vi "SetValue.vi"(0 "class data in":refnum<class "AbruptChange.lvclass">, 5 "Value":dbl, 11 "error in (no error)":errorcluster) -> (4 "class data out":refnum<class "AbruptChange.lvclass">, 15 "error out":errorcluster)   [LabVIEW 2019, in "AbruptChange.lvclass"]
uses:
  AbruptChange.lvclass
  AbruptChange.lvclass/AbruptChange.ctl
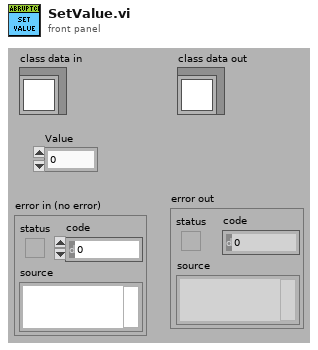
[diagram p1: front panel]
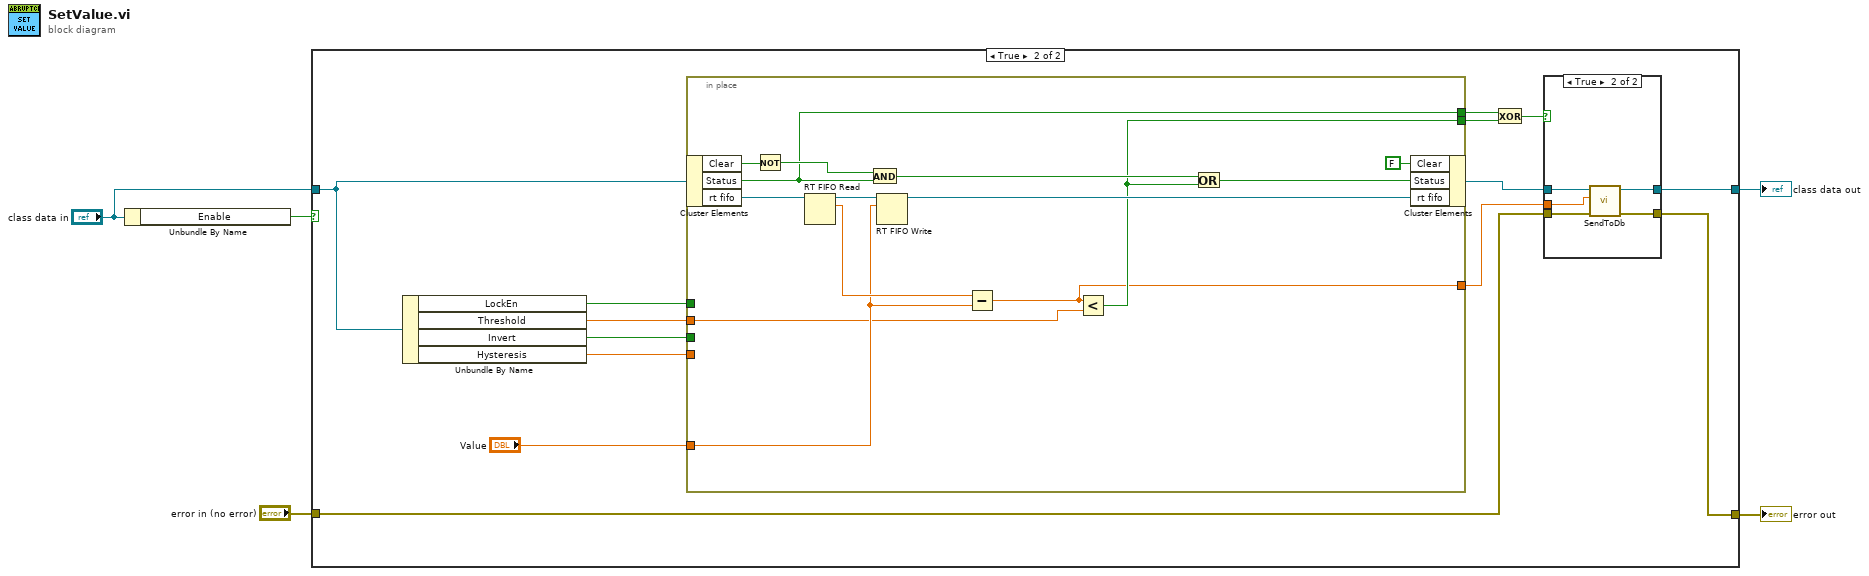
[diagram p0: block diagram]
diagram:
  n1 = Unbundle By Name("class data in") -> ("Enable"=w4:bool)
  n2 = case shown="True" w4 {
    tunnel: [w7 w15] -> w5
    tunnel: "class data in" -> [w7 w21]
    tunnel: "error in (no error)" -> [w6 w14]
    tunnel: [w6 w13] -> w1
    frame False {
    }
    frame True {
      n3 = Unbundle By Name(w21) -> ("LockEn"=w17:bool, "Threshold"=w19:dbl, "Invert"=w18:bool, "Hysteresis"=w20:dbl)
      n4 = in-place {
        in-place-border: w19 -> [w38]
        in-place-border: w20 -> [_]
        in-place-border: w18 -> [_]
        in-place-border: w17 -> [_]
        in-place-border: "Value" -> [w39]
        in-place-border: [w31] -> w10
        in-place-border: [w30] -> w9
        in-place-border: [w29] -> w8
        n5 = in-place-cluster #1(w21) -> ("Clear"=w34:bool, "Status"=w30:bool, "rt fifo"=w42:refnum<k33>)
        n6 = Not(x=w34) -> (.not. x?=w35:bool)
        n7 = RT FIFO Read(0:w42) -> (8:w41:refnum<k33>, 9:w40:dbl)  [unwired: 3 in, 3 out]
        n8 = And(x=w35, y=w30) -> (x .and. y?=w36:bool)
        n9 = RT FIFO Write(0:w41, 1:w39) -> (8:w37:refnum<k33>)  [unwired: 3 in, 3 out]
        n10 = Subtract(x=w40, y=w39) -> (x-y=w29:dbl)
        n11 = Less?(x=w29, y=w38) -> (x < y?=w31:bool)
        n12 = Or(x=w36, y=w31) -> (x .or. y?=w33:bool)
        n13 = in-place-cluster #1("Clear"=FALSE, "Status"=w33, "rt fifo"=w37) -> (w16:refnum<class "AbruptChange.lvclass">)
      }
      n14 = Exclusive Or(1:w10, 2:w9) -> (0:w12:bool)
      n15 = case shown="True" w12 {
        tunnel: w16 -> [w23 w28]
        tunnel: [w23 w27] -> w15
        tunnel: w14 -> [w22 w26]
        tunnel: [w22 w25] -> w13
        tunnel: w8 -> [_ w24]
        frame False {
        }
        frame True {
          n16 = call "SendToDb.vi"("error in (no error)"=w26, "Value DBL"=w24, "AnalogComparator in"=w28) -> ("error out"=w25:errorcluster, "AnalogComparator out"=w27:refnum<class "AbruptChange.lvclass">)  [unwired: 7 in]
        }
      }
    }
  }
  "class data out" <- w5
  "error out" <- w1
